vi "Diagonal.vi"(1 "Diagonal":T1 items=["0", "45", "90", "135", "180", "225", "270", "315"]) -> (0 "Diagonal":bool)   [LabVIEW 2014]
uses:
  Controls/Direction enum.ctl
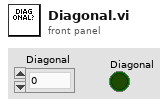
[diagram p1: front panel]
types:
  T1 = typedef "Direction enum.ctl" = u16
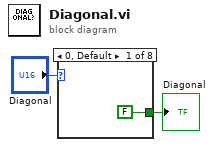
[diagram p0: block diagram]
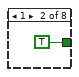
[diagram p2: hidden frame]
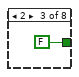
[diagram p3: hidden frame]
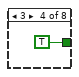
[diagram p4: hidden frame]
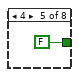
[diagram p5: hidden frame]
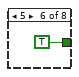
[diagram p6: hidden frame]
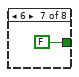
[diagram p7: hidden frame]
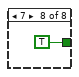
[diagram p8: hidden frame]
diagram:
  n1 = case shown="0, Default" "Diagonal" {
    tunnel: [FALSE TRUE FALSE TRUE FALSE TRUE FALSE TRUE] -> w1
    frame 0, Default {
    }
    frame 1 {
    }
    frame 2 {
    }
    frame 3 {
    }
    frame 4 {
    }
    frame 5 {
    }
    frame 6 {
    }
    frame 7 {
    }
  }
  "Diagonal" <- w1
